vi "NanotecSMCPDDriver.move absolute.vi"(0 "VISA resource name":refnum<visa-resource-name>, 1 "contollerID":i32=-1, 3 "nOfSteps [uSteps]":i32, 5 "error in (no error)":errorcluster) -> (14 "VISA resource name out":refnum<visa-resource-name>, 15 "contollerID out":i32=-1, 19 "error out":errorcluster)   [LabVIEW 2014, in "NanotecSMCPDDriver.lvlib"]
doc: "Performs a movement to the requested absolute position. When using this VI, the controller should be in state \"ready\". This VI just starts the movement. It does not wait until the final position is reached."
uses:
  NanotecSMCPDDriver.lvlib
  Private/NanotecSMCPDDriver.positioning mode types.ctl
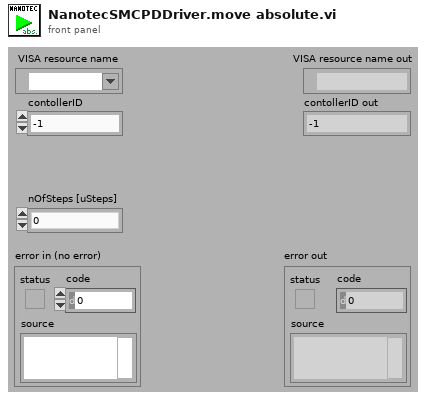
[diagram p1: front panel]
types:
  T1 = typedef "NanotecSMCPDDriver.lvlib/NanotecSMCPDDriver.positioning mode types.ctl" = enum16{"unknown", "relative positioning", "absolute positioning", "internal referencing", "external referencing"}
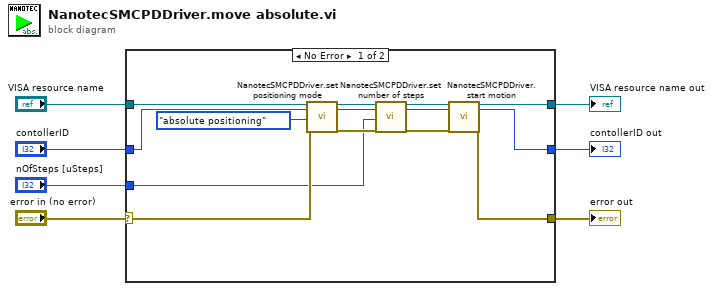
[diagram p0: block diagram]
diagram:
  n1 = case shown="No Error" "error in (no error)" {
    selector: "error in (no error)" -> [w12 w22]
    tunnel: [w18 w24] -> w7
    tunnel: [w13 w22] -> w6
    tunnel: "VISA resource name" -> [w21 w24]
    tunnel: "contollerID" -> [w17 w23]
    tunnel: [w14 w23] -> w3
    tunnel: "nOfSteps [uSteps]" -> [w9 _]
    frame No Error {
      n2 = call "NanotecSMCPDDriver.set positioning mode.vi"("VISA resource name"=w21, "contollerID"=w17, "positioningMode"=NanotecSMCPDDriver.positioning_mode_types."absolute positioning", "error in (no error)"=w12) -> ("VISA resource name out"=w20:refnum<visa-resource-name>, "contollerID out"=w16:i32, "error out"=w11:errorcluster)  [unwired: 13 in]
      n3 = call "NanotecSMCPDDriver.set number of steps.vi"("VISA resource name"=w20, "contollerID"=w16, "nOfSteps [uSteps]"=w9, "error in (no error)"=w11) -> ("VISA resource name out"=w19:refnum<visa-resource-name>, "contollerID out"=w15:i32, "error out"=w10:errorcluster)  [unwired: 13 in]
      n4 = call "NanotecSMCPDDriver.start motion.vi"("VISA resource name"=w19, "contollerID"=w15, "error in (no error)"=w10) -> ("VISA resource name out"=w18:refnum<visa-resource-name>, "contollerID out"=w14:i32, "error out"=w13:errorcluster)  [unwired: 14 in]
    }
    frame Error {
    }
  }
  "VISA resource name out" <- w7
  "error out" <- w6
  "contollerID out" <- w3
